vi "ixon setup FT acquisition 2.vi"(6 "EM CCD Gain":u16(slide)=230 scale=0.01..255.0, 7 "Interactive?":bool=TRUE, 8 "error in (no error)":errorcluster, 9 "Exposure Time (sec)":sgl(slide)=0.1 scale=0.001..10.0 scale format="%#_1g", 10 "Readout Settings":T1={"Acquisition Mode"=enum."Frame Transfer Run till Abort", "Pixel Rate"=enum."EM CCD 20 Mhz 16 bits", "High Capacity?"=FALSE, "V Shift Speed (us/row)"=enum."4.33", "V Shift Amplitude"=enum."normal", "Preamp Gain"=enum."1", "Trigger Mode"=0, "Baseline offset"=0, "Baseline clamp"=FALSE} {"Baseline offset" min=-1000 max=1000 step=100; "Trigger Mode" items=["Internal", "External"]}, 11 "Image Size":T3={"H Bin"=1, "V Bin"=1, "Left"=1, "Top"=1, "Right"=512, "Bottom"=512}) -> (0 "error out":errorcluster, 1 "Actual Image Height":i32, 2 "Actual Image Width":i32, 3 "Actual Exposure Time (sec)":sgl format="%.4f")   [LabVIEW 2016]
doc: "Programs the hardware settings into the Andor iXon camera and prepares it for acquisition. This VI is currently designed for use with the \"Frame Transfer Run till Abort\" acquisition mode; it has not been tested with other modes."
uses:
  ixon ultra 897/ixon readout settings.ctl
  ixon ultra 897/andor acquisition mode.ctl
  <userlib>/atmcd32d.llb/Shutter_type typedef.ctl
  ixon ultra 897/HAL Camera specifications globals.vi
  ATMCD32D.DLL
panel:
  in  "Cancel":bool
  in  "Program Camera":bool
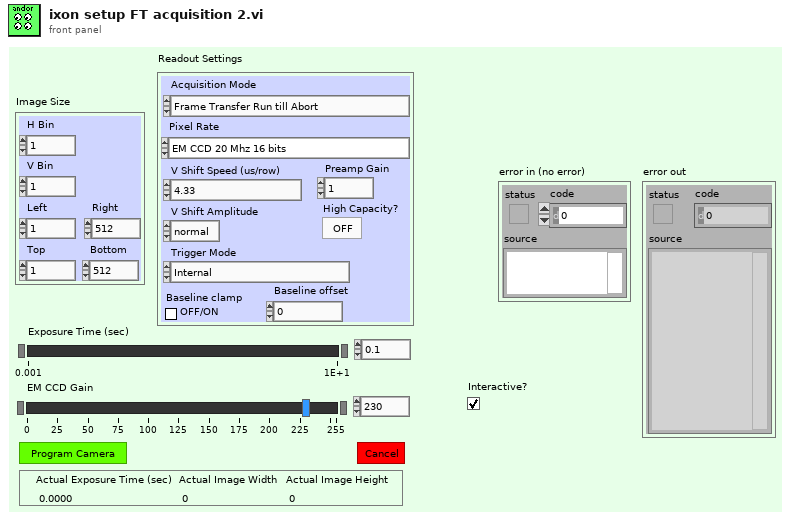
[diagram p1: front panel]
types:
  T1 = typedef "ixon readout settings.ctl" = cluster{"Acquisition Mode":T2, "Pixel Rate":enum16{"EM CCD 30 Mhz 16 bits", "EM CCD 20 Mhz 16 bits", "EM CCD 10 Mhz 16 bits", "EM CCD 1 Mhz 16 bits", "Standard CCD 1 Mhz 16 bits", "Standard CCD 0.1 Mhz 16 bits"}, "High Capacity?":bool, "V Shift Speed (us/row)":enum16{"0.6 (not reccommended)", "1.13  (not reccommended)", "2.2  (not reccommended)", "4.33"}, "V Shift Amplitude":enum16{"normal", "+1", "+2", "+3", "+4"}, "Preamp Gain":enum16{"1", "2", "3"}, "Trigger Mode":u32, "Baseline offset":i16, "Baseline clamp":bool}
  T2 = typedef "andor acquisition mode.ctl" = enum16{"(do not use)", "Single Scan", "Accumulate", "Kinetics", "Fast Kinetics", "Kinetics Run till Abort", "Frame Transfer", "Frame Transfer Run till Abort", "(do not use) ", "Time Delayed Integration"}
  T3 = cluster{"H Bin":i32, "V Bin":i32, "Left":i32, "Top":i32, "Right":i32, "Bottom":i32}
  T4 = enum16{"EM CCD 30 Mhz 16 bits", "EM CCD 20 Mhz 16 bits", "EM CCD 10 Mhz 16 bits", "EM CCD 1 Mhz 16 bits", "Standard CCD 1 Mhz 16 bits", "Standard CCD 0.1 Mhz 16 bits"}
  T5 = enum16{"0.6 (not reccommended)", "1.13  (not reccommended)", "2.2  (not reccommended)", "4.33"}
  T6 = cluster{"Adc Channel":i32, "H Shift Setting":i32, "EM on?":bool}[]
  T7 = cluster{"Adc Channel":i32, "H Shift Setting":i32, "EM on?":bool}
  T8 = typedef "Shutter_type typedef.ctl" = enum16{"TTL Low", "TTL High"}
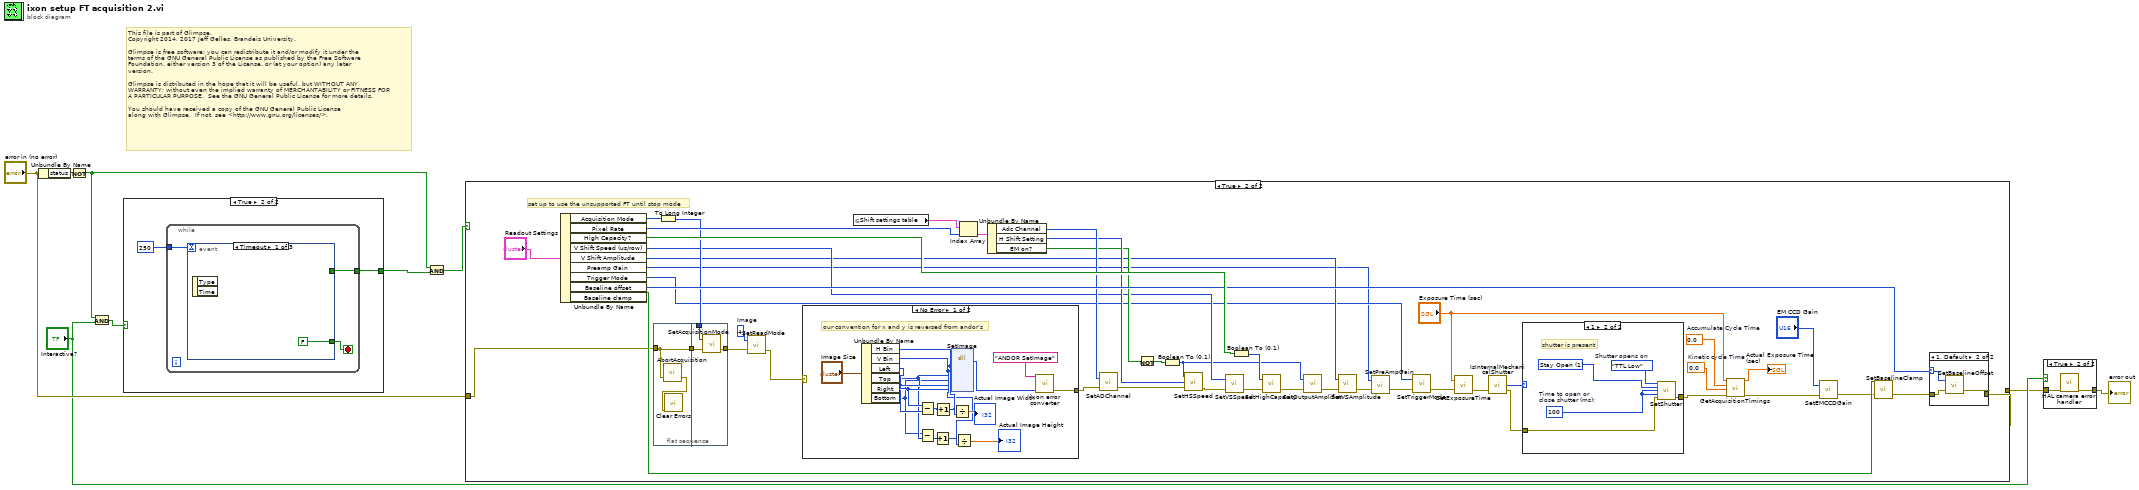
[diagram p0: block diagram]
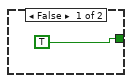
[diagram p6: hidden frame]
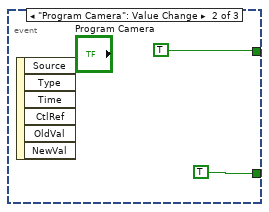
[diagram p7: hidden frame]
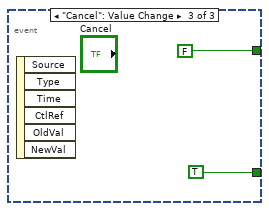
[diagram p8: hidden frame]
diagram:
  # "This file is part of Glimpse. \nCopyright 2014, 2017 Jeff Gelles, Brandeis University.    \n\nGlimpse is free software: you can redistribute it and/or modify it under the \nterms of the GNU General Public License as published by the Free Software \nFoundation, either version 3 of the License, or (at your option) any later \nversion.\n\nGlimpse is distributed in the hope that it will be useful, but WITHOUT ANY \nWARRANTY; without even the implied warranty of MERCHANTABILITY or FITNESS FOR \nA PARTICULAR PURPOSE.  See the GNU General Public License for more details.\n\nYou should have received a copy of the GNU General Public License\nalong with Glimpse.  If not, see <http://www.gnu.org/licenses/>."
  n1 = Unbundle By Name("error in (no error)") -> ("status"=w9:bool)
  n2 = Not(x=w9) -> (.not. x?=w5:bool)
  n3 = And(x=w5, y="Interactive?") -> (x .and. y?=w8:bool)
  n4 = case shown="True" w8 {
    tunnel: [TRUE w11] -> w7
    frame False {
    }
    frame True {
      n5 = while {
        tunnel: 250 -> [w15]
        tunnel: [w14] -> w11
        stop <- w13 stop-if-true
        n6 = event shown="[0] Timeout" {
          selector: _ -> [_ _ _]
          dyn-events: _ -> [_ _ _]
          timeout: w15 -> [_ _ _]
          tunnel: [_ TRUE FALSE] -> w14
          tunnel: [FALSE TRUE TRUE] -> w13
          event Timeout {
            n7 = event-data() -> ()  [unwired: 3 out]
          }
          event "Program Camera": Value Change {
            n8 = event-data() -> ()  [unwired: 7 out]
          }
          event "Cancel": Value Change {
            n9 = event-data() -> ()  [unwired: 7 out]
          }
        }
      }
    }
  }
  n10 = And(x=w5, y=w7) -> (x .and. y?=w6:bool)
  n11 = case shown="True" w6 {
    tunnel: [w21 w67] -> w2
    tunnel: "error in (no error)" -> [w21 w23]
    frame False {
    }
    frame True {
      w30 = sgl 0.0  # Accumulate Cycle Time
      w31 = sgl 0.0  # Kinetic cycle Time
      w54 = u16 4  # Image
      # "set up to use the unsupported FT until stop mode"
      n12 = Unbundle By Name("Readout Settings") -> ("Acquisition Mode"=w57:T2, "Pixel Rate"=w64:T4, "High Capacity?"=w63:bool, "V Shift Speed (us/row)"=w46:T5, "V Shift Amplitude"=w39:enum16{"normal", "+1", "+2", "+3", "+4"}, "Preamp Gain"=w34:enum16{"1", "2", "3"}, "Trigger Mode"=w37:u32, "Baseline offset"=w59:i16, "Baseline clamp"=w62:bool)
      n13 = flat-sequence {
        tunnel: w23 -> [w69]
        tunnel: [w69] -> w22
        tunnel: w56 -> [w72]
        tunnel: [w71] -> w55
        tunnel: w22 -> [w70]
        frame #0 {
          n14 = call <userlib>:"AbortAcquisition.vi"("error in (no error)"=w69) -> ("error out"=w68:errorcluster)  [unwired: 1 in, 1 out]
          n15 = call <vilib>:"Clear Errors.vi"("error in (no error)"=w68) -> ()  [unwired: 5 in, 2 out]
        }
        frame #1 {
          n16 = call <userlib>:"SetAcquisitionMode.vi"("error in (no error)"=w70, "mode"=w72) -> ("error out"=w71:errorcluster)  [unwired: 1 out]
        }
      }
      n17 = To Long Integer(number=w57) -> (32bit integer=w56:i32)
      n18 = call <userlib>:"SetReadMode.vi"("error in (no error)"=w55, "mode"=w54) -> ("error out"=w53:errorcluster)  [unwired: 1 out]
      n19 = case shown="No Error" w53 {
        selector: w53 -> [_ w89]
        tunnel: [w86 w89] -> w52
        frame No Error {
          # "our convention for x and y is reversed from andor's"
          n20 = Unbundle By Name("Image Size") -> ("H Bin"=w82:i32, "V Bin"=w80:i32, "Left"=w75:i32, "Top"=w74:i32, "Right"=w76:i32, "Bottom"=w73:i32)
          n21 = Subtract(x=w76, y=w75) -> (x-y=w83:i32)
          n22 = Subtract(x=w73, y=w74) -> (x-y=w81:i32)
          n23 = Increment(x=w81) -> (x+1=w77:i32)
          n24 = Increment(x=w83) -> (x+1=w78:i32)
          n25 = dll-call lib="Atmcd32d.dll" fn="SetImage"(w82, w80, w74, w73, w75, w76) -> (w87:u32)  [unwired: 9 in, 2 out]
          n26 = Divide(x=w78, y=w82) -> (x/y=→"Actual Image Width":dbl)
          n27 = Divide(x=w77, y=w80) -> (x/y=→"Actual Image Height":dbl)
          n28 = call "ixon error converter.vi"("Andor error code"=w87, "source"="ANDOR SetImage") -> ("error out"=w86:errorcluster)  [unwired: 5 out]
        }
        frame Error {
        }
      }
      n29 = global read "HAL Camera specifications globals.vi" "Shift settings table"() -> (w58:T6)
      n30 = Index Array(array=w58, index=w64) -> (element=w66:T7)
      n31 = Unbundle By Name(w66) -> ("Adc Channel"=w51:i32, "H Shift Setting"=w50:i32, "EM on?"=w49:bool)
      n32 = call <userlib>:"SetADChannel.vi"("error in (no error)"=w52, "channel"=w51) -> ("error out"=w47:errorcluster)  [unwired: 1 out]
      n33 = Not(x=w49) -> (.not. x?=w48:bool)
      n34 = Boolean To (0,1)(Boolean=w48) -> (0, 1=w42:i16)
      n35 = call <userlib>:"SetHSSpeed.vi"("error in (no error)"=w47, "index"=w50, "type"=w42) -> ("error out"=w45:errorcluster)  [unwired: 1 in, 1 out]
      n36 = call <userlib>:"SetVSSpeed.vi"("error in (no error)"=w45, "index"=w46) -> ("error out"=w44:errorcluster)  [unwired: 1 out]
      n37 = Boolean To (0,1)(Boolean=w63) -> (0, 1=w43:i16)
      n38 = call <userlib>:"SetHighCapacity.vi"("error in (no error)"=w44, "state"=w43) -> ("error out"=w41:errorcluster)  [unwired: 1 out]
      n39 = call <userlib>:"SetOutputAmplifier.vi"("error in (no error)"=w41, "type"=w42) -> ("error out"=w40:errorcluster)  [unwired: 1 out]
      n40 = call <userlib>:"SetVSAmplitude.vi"("error in (no error)"=w40, "amplitude"=w39) -> ("error out"=w38:errorcluster)  [unwired: 1 out]
      n41 = call <userlib>:"SetPreAmpGain.vi"("error in (no error)"=w38, "index"=w34) -> ("error out"=w36:errorcluster)  [unwired: 1 out]
      n42 = call <userlib>:"SetTriggerMode.vi"("error in (no error)"=w36, "mode"=w37) -> ("error out"=w35:errorcluster)  [unwired: 1 out]
      n43 = call <userlib>:"SetExposureTime.vi"("error in (no error)"=w35, "time"="Exposure Time (sec)") -> ("error out"=w33:errorcluster)  [unwired: 1 out]
      n44 = call <userlib>:"IsInternalMechanicalShutter.vi"("error in (no error)"=w33) -> ("error out"=w32:errorcluster, "InternalShutter"=w61:i32)  [unwired: 2 in, 1 out]
      n45 = case shown="1" w61 {
        tunnel: [w90 w95] -> w29
        tunnel: w32 -> [w90 w94]
        frame 0, Default {
        }
        frame 1 {
          w91 = 1 items=["Auto", "Stay Open", "Always Closed"] ("Shutter")
          w93 = Shutter_type_typedef."TTL Low"  # Shutter opens on
          w92 = 100  # Time to open or close shutter (ms):
          # "shutter is present"
          n46 = call <userlib>:"SetShutter.vi"("type"=w93, "mode"=w91, "closingtime"=w92, "openingtime"=w92, "error in (no error)"=w94) -> ("error out"=w95:errorcluster)  [unwired: 9 in, 1 out]
        }
      }
      n47 = call <userlib>:"GetAcquisitionTimings.vi"("exposure input"="Exposure Time (sec)", "accumulate input"=w30, "kinetic input"=w31, "error in (no error)"=w29) -> ("exposure"=→"Actual Exposure Time (sec)":sgl, "error out"=w25:errorcluster)  [unwired: 7 in, 3 out]
      n48 = call <userlib>:"SetEMCCDGain.vi"("error in (no error)"=w25, "gain"="EM CCD Gain") -> ("error out"=w24:errorcluster)  [unwired: 1 out]
      n49 = call <userlib>:"SetBaselineClamp.vi"("error in (no error)"=w24, "state"=w62) -> ("error out"=w60:errorcluster)  [unwired: 1 out]
      n50 = case shown="1, Default" w59 {
        selector: w59 -> [_ w97]
        tunnel: [w96 w98] -> w67
        tunnel: w60 -> [w96 w99]
        frame 0 {
        }
        frame 1, Default {
          n51 = call <userlib>:"SetBaselineOffset.vi"("error in (no error)"=w99, "offset"=w97) -> ("error out"=w98:errorcluster)  [unwired: 1 out]
        }
      }
    }
  }
  n52 = case shown="True" "Interactive?" {
    tunnel: w2 -> [w100 w102]
    tunnel: [w100 w101] -> w1
    frame False {
    }
    frame True {
      n53 = call "HAL camera error handler.vi"("error in (no error)"=w102) -> ("error out"=w101:errorcluster)  [unwired: 10 in]
    }
  }
  "error out" <- w1
